vi "Read Transient Response Time.vi"(8 "error in (no error)":errorcluster, 9 "Source 2 (1: Channel 2)":u16(ring)=1 items=["Channel 1", "Channel 2", "Channel 3", "Channel 4", "Function 1", "Function 2", "Function 3", "Function 4", "Math 1", "Math 2", "Math 3", "Math 4", "Waveform Memory 1", "Waveform Memory 2"], 10 "Source 1 (0: Channel 1)":u16(ring) items=["Channel 1", "Channel 2", "Channel 3", "Channel 4", "Function 1", "Function 2", "Function 3", "Function 4", "Math 1", "Math 2", "Math 3", "Math 4", "Waveform Memory 1", "Waveform Memory 2"], 11 "VISA resource name":refnum<visa-resource-name>) -> (0 "error out":errorcluster, 2 "Transient Response Time":dbl, 3 "VISA resource name out":refnum<visa-resource-name>)   [LabVIEW 2015, in "Agilent 2000 3000 X-Series.lvlib"]
doc: "Returns transient response time measurement result."
uses:
  Agilent 2000 3000 X-Series.lvlib
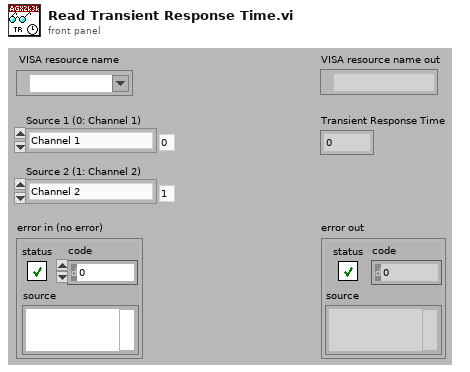
[diagram p1: front panel]
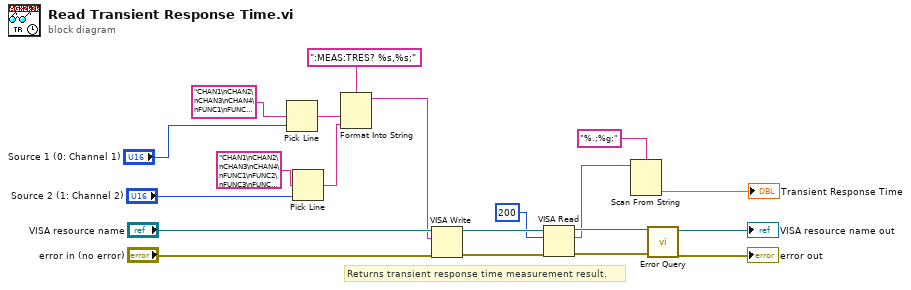
[diagram p0: block diagram]
diagram:
  # "Returns transient response time measurement result."
  n1 = Pick Line(multi-line string="CHAN1\nCHAN2\nCHAN3\nCHAN4\nFUNC1\nFUNC2\nFUNC3\nFUNC4\nMATH1\nMATH2\nMATH3\nMATH4\nWMEM1\nWMEM2", line index="Source 1 (0: Channel 1)") -> (output string=w6:string)  [unwired: 1 in]
  n2 = Pick Line(multi-line string="CHAN1\nCHAN2\nCHAN3\nCHAN4\nFUNC1\nFUNC2\nFUNC3\nFUNC4\nMATH1\nMATH2\nMATH3\nMATH4\nWMEM1\nWMEM2", line index="Source 2 (1: Channel 2)") -> (output string=w5:string)  [unwired: 1 in]
  n3 = Format Into String(format string=":MEAS:TRES? %s,%s;", w6, w5) -> (resulting string=w1:string)  [unwired: 2 in, 1 out]
  n4 = VISA Write(VISA resource name="VISA resource name", write buffer=w1, error in (no error)="error in (no error)") -> (VISA resource name out=w16:refnum<visa-resource-name>, error out=w15:errorcluster)  [unwired: 1 out]
  n5 = VISA Read(VISA resource name=w16, byte count=u32 200, error in (no error)=w15) -> (VISA resource name out=w13:refnum<visa-resource-name>, read buffer=w10:string, error out=w12:errorcluster)  [unwired: 1 out]
  n6 = Scan From String(format string="%.;%g;", input string=w10) -> (output 1=→"Transient Response Time":dbl)  [unwired: 2 in, 4 out]
  n7 = call "Error Query.vi"("error in (no error)"=w12, "VISA resource name"=w13) -> ("error out"=→"error out":errorcluster, "VISA resource name out"=→"VISA resource name out":refnum<visa-resource-name>)  [unwired: 8 out]
